vi "getOrientationFromFile.vi"(9 "currentChannels":string[](array[string]), 11 "Raw data file":path) -> (1 "Probe:Euler:Angles":T1, 2 "Omniprobe:Orientation":string)   [LabVIEW 2021]
uses:
  eulerAngles.ctl
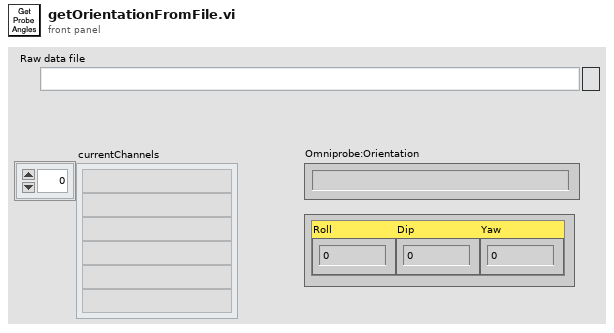
[diagram p1: front panel]
types:
  T1 = typedef "eulerAngles.ctl" = cluster{"Roll":dbl, "Dip":dbl, "Yaw":dbl}
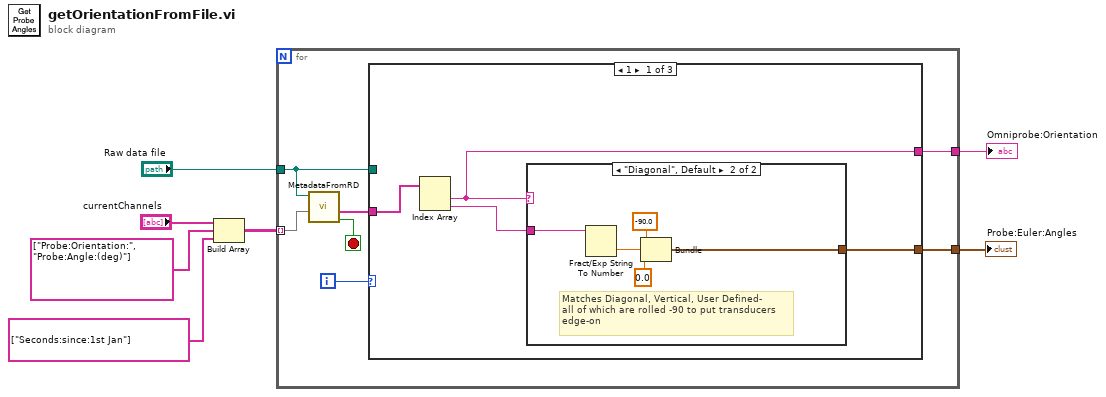
[diagram p0: block diagram]
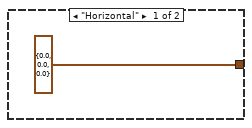
[diagram p2: hidden frame]
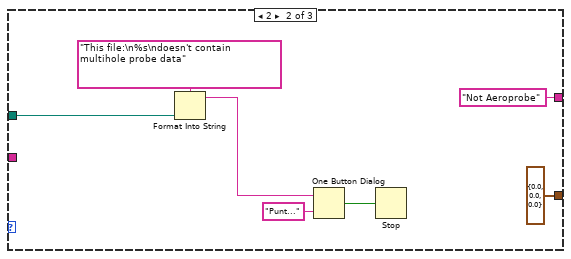
[diagram p3: hidden frame]
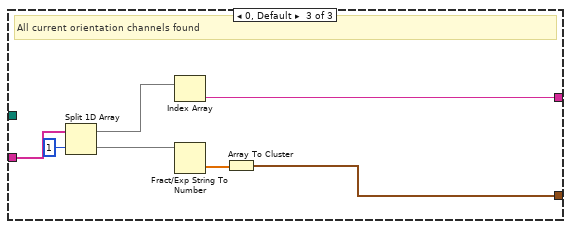
[diagram p4: hidden frame]
diagram:
  n1 = Build Array("currentChannels", string[] ["Probe:Orientation:", "Probe:Angle:(deg)"], string[] ["Seconds:since:1st Jan"]) -> (w2:string[][])
  n2 = for {
    tunnel: "Raw data file" -> [w8]
    tunnel: [w13] -> w6
    tunnel: [w12] -> w5
    tunnel: w2 -> [w11] mode=indexing
    i -> [w10]
    stop <- w9 stop-if-true
    n3 = call "MetadataFromRD.vi"("ChannelNames"=w11, "Raw data file"=w8) -> ("allFound"=w9:bool, "ValueStrings"=w14:string[])  [unwired: 6 in, 2 out]
    n4 = case shown="1" w10 {
      tunnel: w14 -> [w18 _ w38]
      tunnel: [w15 cluster{"[0]":dbl, "[1]":dbl, "[2]":dbl} {"[0]"=0.0, "[1]"=0.0, "[2]"=0.0} w34] -> w13
      tunnel: [w17 "Not Aeroprobe" ("String") w32] -> w12
      tunnel: w8 -> [_ w27 _]
      frame 1 {
        n5 = Index Array(array=w18) -> (element #1=w17:string, element #2=w16:string)  [unwired: 2 in]
        n6 = case shown="\"Diagonal\", Default" w17 {
          tunnel: w16 -> [_ w24]
          tunnel: [cluster{"[0]":dbl, "[1]":dbl, "[2]":dbl} {"[0]"=0.0, "[1]"=0.0, "[2]"=0.0} w20] -> w15
          frame "Horizontal" {
          }
          frame "Diagonal", Default {
            # "Matches Diagonal, Vertical, User Defined-\nall of which are rolled -90 to put transducers edge-on"
            n7 = Fract/Exp String To Number(string=w24) -> (number=w22:dbl)  [unwired: 3 in, 1 out]
            n8 = Bundle(-90.0, w22, 0.0) -> (w20:cluster{dbl, dbl, dbl})  [unwired: 1 in]
          }
        }
      }
      frame 2 {
        n9 = Format Into String(format string="This file:\n%s\ndoesn't contain multihole probe data" ("message"), w27) -> (resulting string=w26:string)  [unwired: 2 in, 1 out]
        n10 = One Button Dialog(message=w26, button name ("OK")="Punt...") -> (true=w25:bool)
        n11 = Stop(stop? (T)=w25) -> ()
      }
      frame 0, Default {
        # "All current orientation channels found"
        n12 = Split 1D Array(array=w38, index=1) -> (first subarray=w33:string[], second subarray=w36:string[])
        n13 = Index Array(array=w33) -> (element=w32:string)  [unwired: 1 in]
        n14 = Fract/Exp String To Number(string=w36) -> (number=w35:dbl[])  [unwired: 3 in, 1 out]
        n15 = Array To Cluster(array=w35) -> (cluster=w34:cluster{"[0]":dbl, "[1]":dbl, "[2]":dbl})
      }
    }
  }
  "Probe:Euler:Angles" <- w6
  "Omniprobe:Orientation" <- w5
